vi "Set All Param Areas.vi"   [LabVIEW 2020]
uses:
  <vilib>/Utility/miscctls.llb/LVPositionTypeDef.ctl
panel:
  # "This sets the parameters decoration to a standard size and resets the\nwindow of the VI to the decoration size.  It operates on all templates in\nthe Instruments Directory."
types:
  T1 = typedef "LVPositionTypeDef.ctl" = cluster{"Left":i32, "Top":i32}
  T2 = typedef "LVRectTypeDef.ctl" = cluster{"Left":i16, "Top":i16, "Right":i16, "Bottom":i16}
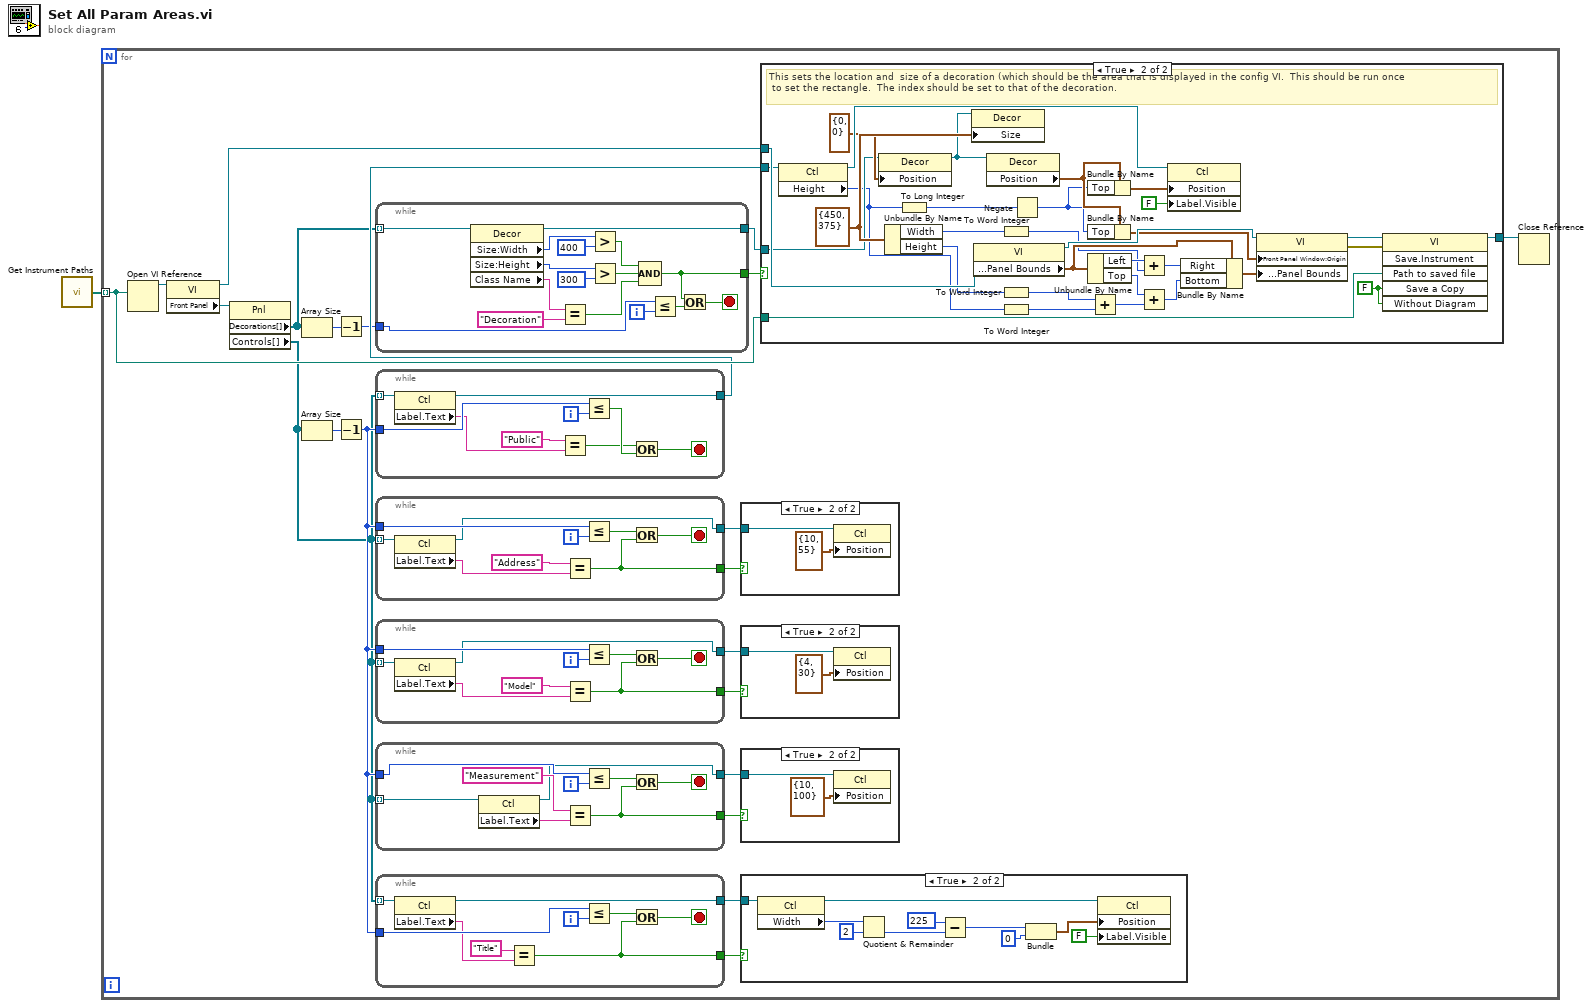
[diagram p0: block diagram]
diagram:
  n1 = call "Get Instrument Paths.vi"() -> ("paths"=w1:path[])  [unwired: 1 in]
  n2 = for {
    tunnel: w1 -> [w19] mode=indexing
    n3 = Open VI Reference(vi path=w19) -> (vi reference=w22:refnum<vi>)  [unwired: 5 in, 1 out]
    n4 = property class="VI"(reference=w22) -> (reference out=w21:refnum<vi>, "Front Panel"=w23:refnum<vi>)  [unwired: 1 in, 1 out]
    n5 = property class="Pnl"(reference=w23) -> ("Decorations[]"=w2:refnum<vi>[], "Controls[]"=w7:refnum<vi>[])  [unwired: 1 in, 2 out]
    n6 = Array Size(array=w2) -> (size(s)=w6:i32)
    n7 = Array Size(array=w7) -> (size(s)=w18:i32)
    n8 = Decrement(x=w6) -> (x-1=w5:i32)
    n9 = Decrement(x=w18) -> (x-1=w10:i32)
    n10 = while {
      tunnel: w5 -> [w86]
      tunnel: [w75] -> w4
      tunnel: [w74] -> w3
      tunnel: w2 -> [w73] mode=indexing
      i -> [w88]
      stop <- w85 stop-if-true
      n11 = property class="Decor"(reference=w73) -> (reference out=w75:refnum<vi>, "Size:Width"=w76:u32, "Size:Height"=w78:u32, "Class Name"=w80:string)  [unwired: 1 in, 1 out]
      n12 = Equal?(x=w80, y="Decoration") -> (x = y?=w84:bool)
      n13 = Greater?(x=w76, y=u32 400) -> (0:w82:bool)
      n14 = Greater?(x=w78, y=u32 300) -> (0:w83:bool)
      n15 = Compound Arithmetic op=AND(w82, w83, w84) -> (w74:bool)
      n16 = Less Or Equal?(x=w86, y=w88) -> (x <= y?=w87:bool)
      n17 = Or(x=w74, y=w87) -> (x .or. y?=w85:bool)
    }
    n18 = while {
      tunnel: w10 -> [w131]
      tunnel: w7 -> [w130] mode=indexing
      tunnel: [w125] -> w17
      i -> [w133]
      stop <- w127 stop-if-true
      n19 = property class="Ctl"(reference=w130) -> (reference out=w125:refnum<vi>, "Label.Text"=w129:string)  [unwired: 1 in, 1 out]
      n20 = Equal?(x="Public", y=w129) -> (x = y?=w126:bool)
      n21 = Less Or Equal?(x=w131, y=w133) -> (x <= y?=w132:bool)
      n22 = Or(x=w126, y=w132) -> (x .or. y?=w127:bool)
    }
    n23 = while {
      tunnel: w10 -> [w113]
      tunnel: w7 -> [w112] mode=indexing
      tunnel: [w108] -> w14
      tunnel: [w107] -> w13
      i -> [w115]
      stop <- w109 stop-if-true
      n24 = property class="Ctl"(reference=w112) -> (reference out=w108:refnum<vi>, "Label.Text"=w111:string)  [unwired: 1 in, 1 out]
      n25 = Equal?(x="Address", y=w111) -> (x = y?=w107:bool)
      n26 = Less Or Equal?(x=w113, y=w115) -> (x <= y?=w114:bool)
      n27 = Or(x=w114, y=w107) -> (x .or. y?=w109:bool)
    }
    n28 = while {
      tunnel: w10 -> [w104]
      tunnel: w7 -> [w103] mode=indexing
      tunnel: [w99] -> w12
      tunnel: [w98] -> w11
      i -> [w106]
      stop <- w100 stop-if-true
      n29 = property class="Ctl"(reference=w103) -> (reference out=w99:refnum<vi>, "Label.Text"=w102:string)  [unwired: 1 in, 1 out]
      n30 = Equal?(x="Model", y=w102) -> (x = y?=w98:bool)
      n31 = Less Or Equal?(x=w104, y=w106) -> (x <= y?=w105:bool)
      n32 = Or(x=w105, y=w98) -> (x .or. y?=w100:bool)
    }
    n33 = while {
      tunnel: w10 -> [w95]
      tunnel: w7 -> [w94] mode=indexing
      tunnel: [w90] -> w9
      tunnel: [w89] -> w8
      i -> [w97]
      stop <- w91 stop-if-true
      n34 = property class="Ctl"(reference=w94) -> (reference out=w90:refnum<vi>, "Label.Text"=w93:string)  [unwired: 1 in, 1 out]
      n35 = Equal?(x="Measurement", y=w93) -> (x = y?=w89:bool)
      n36 = Less Or Equal?(x=w95, y=w97) -> (x <= y?=w96:bool)
      n37 = Or(x=w96, y=w89) -> (x .or. y?=w91:bool)
    }
    n38 = while {
      tunnel: w10 -> [w122]
      tunnel: w7 -> [w121] mode=indexing
      tunnel: [w117] -> w15
      tunnel: [w116] -> w16
      i -> [w124]
      stop <- w118 stop-if-true
      n39 = property class="Ctl"(reference=w121) -> (reference out=w117:refnum<vi>, "Label.Text"=w120:string)  [unwired: 1 in, 1 out]
      n40 = Equal?(x="Title", y=w120) -> (x = y?=w116:bool)
      n41 = Less Or Equal?(x=w122, y=w124) -> (x <= y?=w123:bool)
      n42 = Or(x=w123, y=w116) -> (x .or. y?=w118:bool)
    }
    n43 = case shown="True" w13 {
      tunnel: w14 -> [_ w28]
      frame False {
      }
      frame True {
        n44 = property class="Ctl"(reference=w28, "Position"=T1 {"Left"=10, "Top"=55}) -> ()  [unwired: 1 in, 2 out]
      }
    }
    n45 = case shown="True" w11 {
      tunnel: w12 -> [_ w26]
      frame False {
      }
      frame True {
        n46 = property class="Ctl"(reference=w26, "Position"=T1 {"Left"=4, "Top"=30}) -> ()  [unwired: 1 in, 2 out]
      }
    }
    n47 = case shown="True" w8 {
      tunnel: w9 -> [_ w24]
      frame False {
      }
      frame True {
        n48 = property class="Ctl"(reference=w24, "Position"=T1 {"Left"=10, "Top"=100}) -> ()  [unwired: 1 in, 2 out]
      }
    }
    n49 = case shown="True" w16 {
      tunnel: w15 -> [_ w39]
      frame False {
      }
      frame True {
        n50 = property class="Ctl"(reference=w39) -> (reference out=w38:refnum<vi>, "Width"=w36:u32)  [unwired: 1 in, 1 out]
        n51 = Quotient & Remainder(x=w36, y=u32 2) -> (floor(x/y)=w34:u32)  [unwired: 1 out]
        n52 = Subtract(x=225 ("Left"), y=w34) -> (x-y=w32:u32)
        n53 = Bundle(w32, "Left"=0) -> (w30:cluster{u32, "Left":i32})  [unwired: 1 in]
        n54 = property class="Ctl"(reference=w38, "Position"=w30, "Label.Visible"=FALSE) -> ()  [unwired: 1 in, 2 out]
      }
    }
    n55 = case shown="True" w3 {
      tunnel: w4 -> [_ w47]
      tunnel: w21 -> [w40 w69]
      tunnel: [w40 w70] -> w20
      tunnel: w19 -> [_ w56]
      tunnel: w17 -> [_ w53]
      frame False {
      }
      frame True {
        w45 = FALSE ("Save a Copy")
        w66 = cluster{"Width":u32, "Height":u32} {"Width"=450, "Height"=375} ("Size")
        # "This sets the location and  size of a decoration (which should be the area that is displayed in the config VI.  This should be run once\n to set the rectangle.  The index should be set to that of the decoration."
        n56 = property class="Ctl"(reference=w53) -> (reference out=w51:refnum<vi>, "Height"=w43:u32)  [unwired: 1 in, 1 out]
        n57 = property class="Decor"(reference=w47, "Position"=T1 {"Left"=0, "Top"=0}) -> (reference out=w46:refnum<vi>)  [unwired: 1 in, 1 out]
        n58 = Unbundle By Name(w66) -> ("Width"=w64:u32, "Height"=w61:u32)
        n59 = To Long Integer(number=w43) -> (32bit integer=w42:i32)
        n60 = property class="Decor"(reference=w46, "Size"=w66) -> ()  [unwired: 1 in, 2 out]
        n61 = property class="VI"(reference=w69) -> (reference out=w68:refnum<vi>, "Front Panel Window:Panel Bounds"=w67:T2)  [unwired: 1 in, 1 out]
        n62 = property class="Decor"(reference=w46) -> ("Position"=w49:T1)  [unwired: 1 in, 2 out]
        n63 = To Word Integer(number=w64) -> (16bit integer=w59:i16)
        n64 = To Word Integer(number=w61) -> (16bit integer=w58:i16)
        n65 = To Word Integer(number=w43) -> (16bit integer=w41:i16)
        n66 = Negate(x=w42) -> (-x=w44:i32)
        n67 = Bundle By Name(cluster=w49, "Top"=w44) -> (w52:T1)
        n68 = Bundle By Name(cluster=w49, "Top"=w44) -> (w54:T1)
        n69 = Unbundle By Name(w67) -> ("Left"=w65:i16, "Top"=w62:i16)
        n70 = Add(x=w58, y=w41) -> (x+y=w55:i16)
        n71 = Add(x=w65, y=w59) -> (x+y=w63:i16)
        n72 = Add(x=w62, y=w55) -> (x+y=w60:i16)
        n73 = property class="Ctl"(reference=w51, "Position"=w52, "Label.Visible"=FALSE) -> ()  [unwired: 1 in, 2 out]
        n74 = Bundle By Name(cluster=w67, "Right"=w63, "Bottom"=w60) -> (w57:T2)
        n75 = property class="VI"(reference=w68, "Front Panel Window:Origin"=w54, "Front Panel Window:Panel Bounds"=w57) -> (reference out=w71:refnum<vi>, error out=w72:errorcluster)  [unwired: 1 in]
        n76 = invoke class="VI" method="Save.Instrument"(reference=w71, error in=w72, "Path to saved file"=w56, "Save a Copy"=w45, "Without Diagram"=w45) -> (reference out=w70:refnum<vi>)  [unwired: 1 in, 5 out]
      }
    }
    n77 = Close Reference(reference=w20) -> ()  [unwired: 1 in, 1 out]
  }
